vi "buscaclip.vi"(0 "input cluster":T1, 1 "Channels values 2":i32[](array[numeric]), 2 "vclip":i32[](array[numeric]), 5 "Channels init":i32[](array[numeric])=[2000], 7 "Boolean":bool, 9 "%desviacio":dbl=5.0, 11 "error out 2":errorcluster, 12 "Number points":i32, 13 "slope":dbl) -> (4 "slope 2":dbl, 6 "vclip 2":i32[](array[numeric]), 10 "XY Graph 2":cluster{dbl[], "Best Linear Fit":dbl[]}[](graph), 15 "error out":errorcluster)   [LabVIEW 2009]
uses:
  <vilib>/Utility/NIReport.llb/NI_report.lvclass
  <vilib>/Analysis/NI_AALPro.lvlib
panel:
  out "XY Graph 4":cluster{dbl[], "Best Linear Fit":dbl[]}(graph)
  out "XY Graph 3":cluster{dbl[], i32[]}(graph)
  in  "L1  50% invented":dbl[][](array[numeric])
  in  "L1 min invented":i32[](array[numeric])=[242, 504, 1031, 2128, 3263, 4418, 5634, 6888]
  out "XY Graph":cluster{"Y":dbl[], "Y":dbl[]}[](graph)
  out "L1  50%":dbl[][](array[numeric])=[[182.05332645693656, 181.0458957661739, 182.31328051706822, 182.44384615384615, 179.9591580860661, 183.67138786049767, 183.0415079653926], [383.1443079334591, 380.3408546343534, 383.09068068207546, 382.9081242164992, 377.8888565224893, 386.4745006061593, 384.33733278296165], [789.794916143154, 783.9334435523022, 789.880331635444, 788.1638578058222, 779.1397265900023, 796.380113600458, 792.3805482207972], [1637.2849189817332, 1624.3008579976345, 1635.9791868307739, 1633.4037928039274, 1613.351662874732, 1647.9524154468106, 1640.5214046384517], [2513.43820756283, 2496.681867952526, 2512.120672224883, 2508.5174246445135, 2478.2432072662637, 2532.0838659445626, 2519.7319162836616], [4350.429616233692, 4325.797863663112, 4346.430175185175, 4343.835753463216, 4286.1263991243895, 4381.02010040906, 4360.577157137679], [5321.96395522116, 5291.780098348377, 5317.9835218197695, 5305.673007498198, 5228.362955923682, 5348.7398745375585, 5316.2612416656], [6878.716199794284, 6844.2297782699125, 6886.512941570447, 6849.728580417201, 6743.132495285984, 6910.301756503628, 6900.4988799604525]]
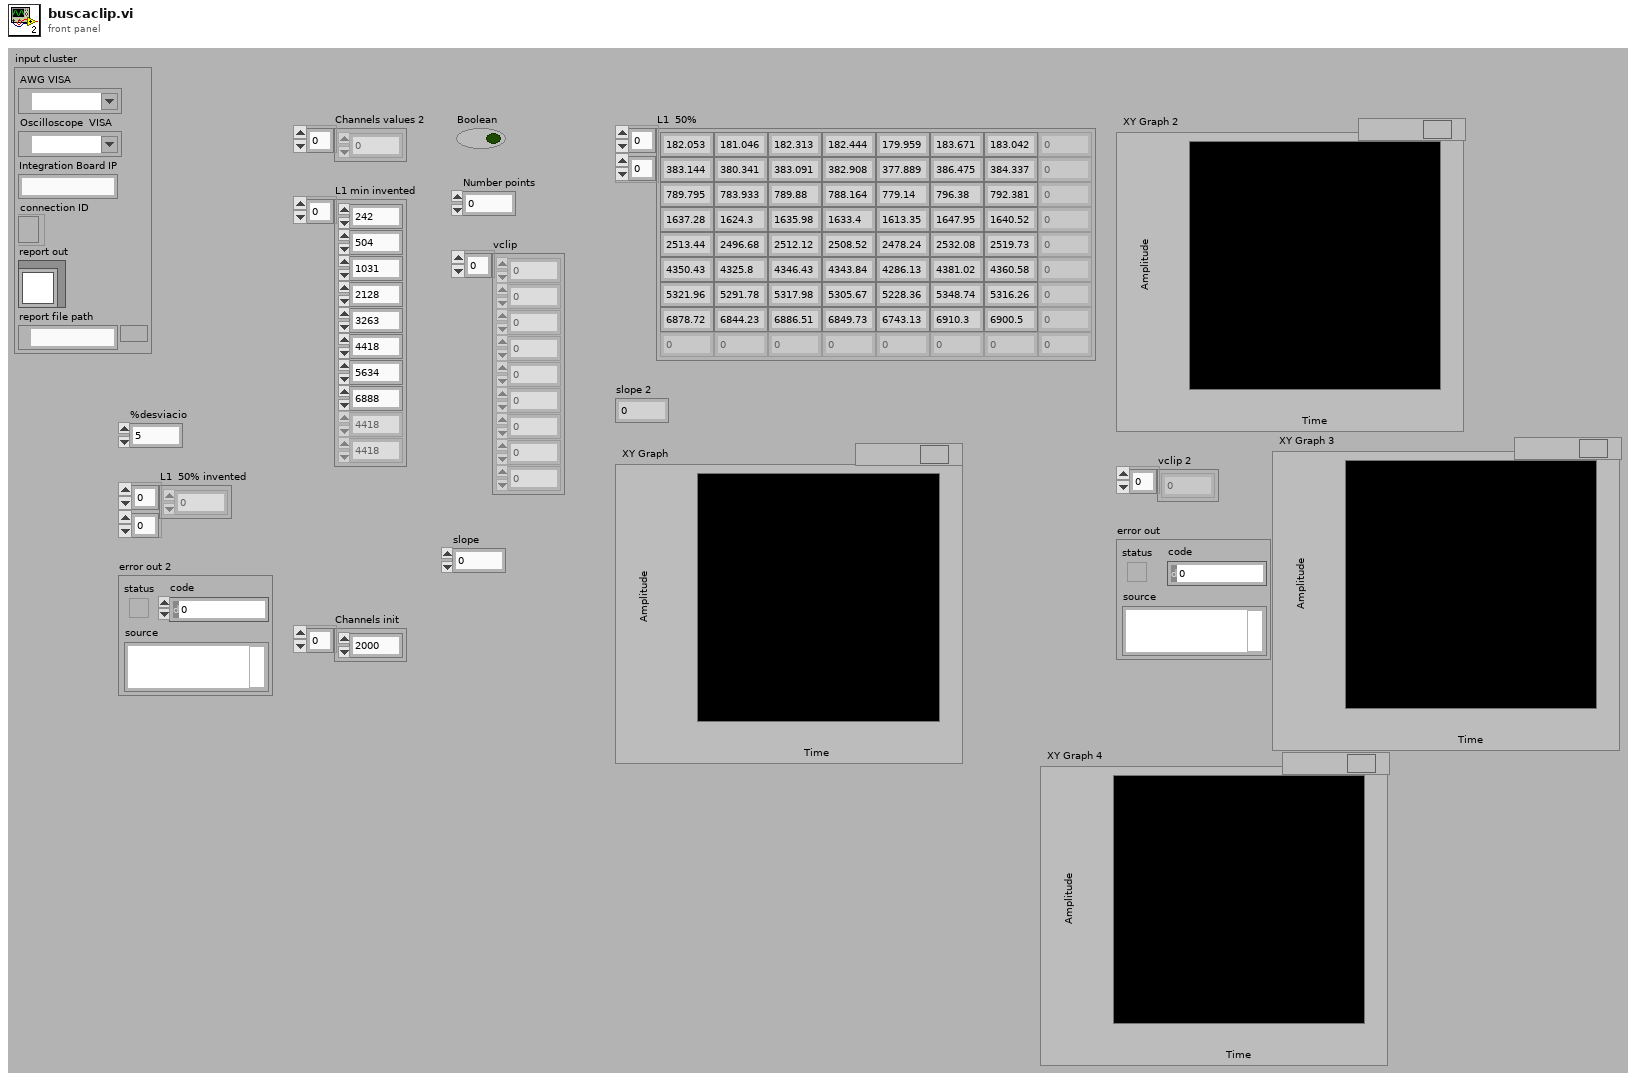
[diagram p1: front panel]
types:
  T1 = cluster{"AWG VISA":refnum<visa-resource-name>, "Oscilloscope  VISA ":refnum<visa-resource-name>, "Integration Board IP":string, "connection ID":refnum<k5>, "report out":refnum<class "NI_report.lvclass">, "report file path":path}
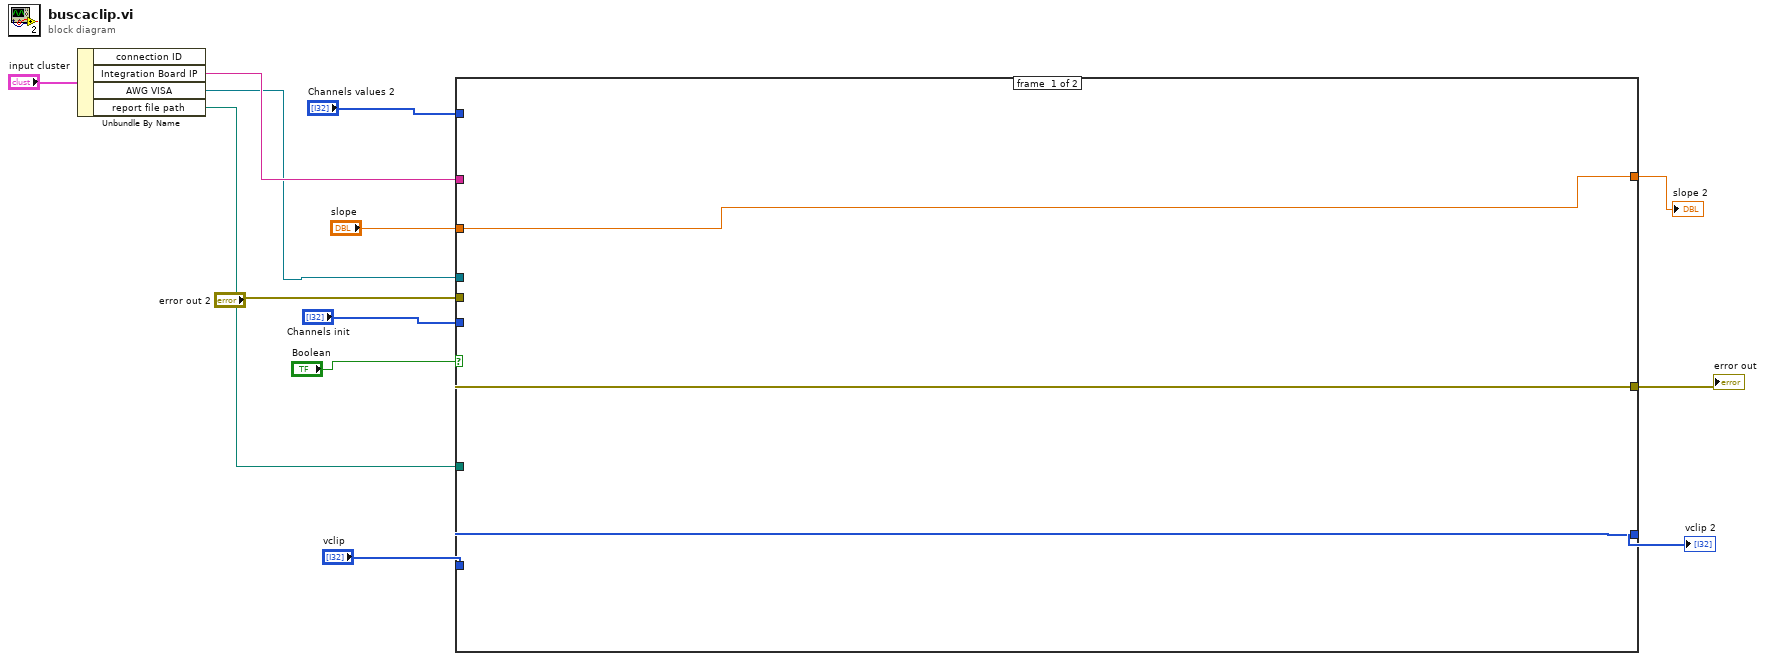
[diagram p0: block diagram]
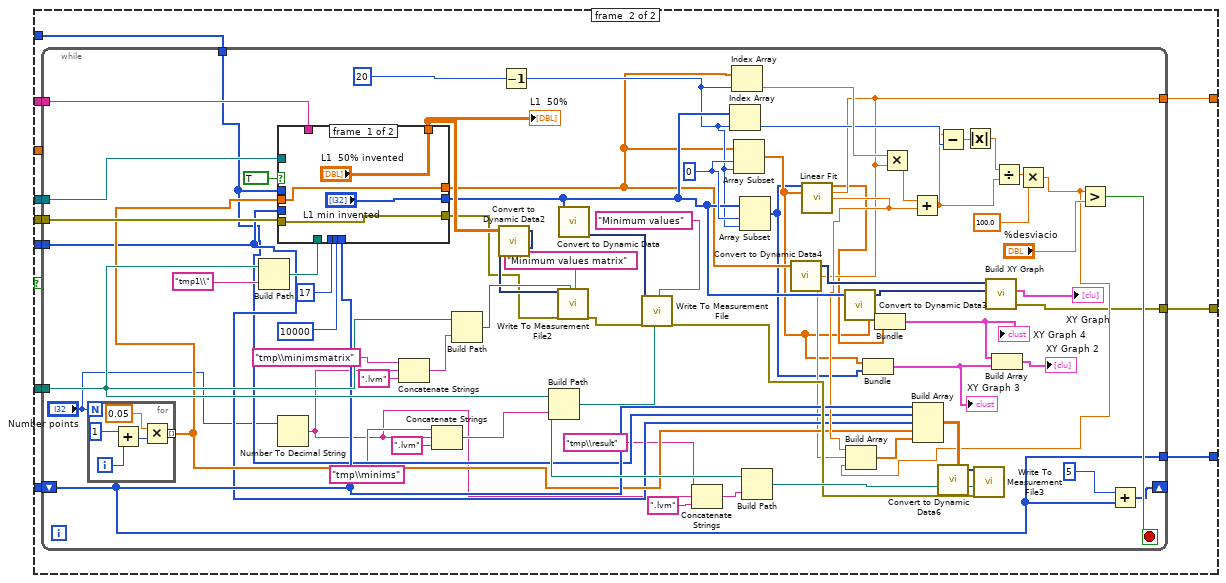
[diagram p2: hidden frame]
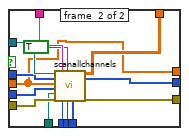
[diagram p3: hidden frame]
diagram:
  n1 = Unbundle By Name("input cluster") -> ("Integration Board IP"=w4:string, "AWG VISA"=w3:refnum<visa-resource-name>, "report file path"=w2:path)  [unwired: 1 out]
  n2 = case shown="True" "Boolean" {
    tunnel: "error out 2" -> [w14 w26]
    tunnel: w3 -> [_ w25]
    tunnel: w4 -> [_ w24]
    tunnel: w2 -> [_ w23]
    tunnel: [w15 w22] -> w11
    tunnel: [w16 w21] -> w7
    tunnel: "vclip" -> [w16 w20]
    tunnel: "Channels init" -> [_ w19]
    tunnel: "Channels values 2" -> [_ w18]
    tunnel: "slope" -> [w15 _]
    tunnel: [w14 w17] -> w13
    frame #0 {
    }
    frame #1 {
      n3 = while {
        tunnel: w26 -> [w91]
        tunnel: w25 -> [w90]
        tunnel: w24 -> [w89]
        tunnel: w23 -> [w62]
        shift-right: [w63] -> _
        shift-left: w20 -> [w59]
        tunnel: [w49] -> w22
        tunnel: [w59] -> w21
        tunnel: w19 -> [w51]
        tunnel: w18 -> [w50]
        tunnel: [w38] -> w17
        stop <- w73 stop-if-true
        w79 = 0 ("length")
        n4 = for {
          N: "Number points" -> [_]
          tunnel: [w95] -> w53 mode=indexing
          i -> [w99]
          n5 = Add(x=1, y=w99) -> (x+y=w97:i32)
          n6 = Multiply(x=0.05 ("y"), y=w97) -> (x*y=w95:dbl)
        }
        n7 = Build Path(base path=w62, name or relative path="tmp1\\") -> (appended path=w87:path)
        n8 = case shown="True" TRUE {
          tunnel: [w103 w117] -> w81
          tunnel: w91 -> [w103 w116]
          tunnel: w90 -> [_ w115]
          tunnel: w89 -> [_ w114]
          tunnel: w51 -> [_ w113]
          tunnel: w53 -> [w100 w104]
          tunnel: w50 -> [_ w112]
          tunnel: 17 ("Value") -> [_ w111]
          tunnel: 10000 ("Value") -> [_ w110]
          tunnel: ["L1 min invented" w108] -> w65
          tunnel: w87 -> [_ w107]
          tunnel: w59 -> [_ w106]
          tunnel: ["L1  50% invented" w105] -> w83
          tunnel: [w100 w104] -> w33
          frame #0 {
          }
          frame #1 {
            n9 = call "scanallchannels.vi"("VISA resource name out"=w115, "nm ch"=w112, "Voltages values"=w104, "Init ch value"=w113, "base path"=w107, "error in"=w116, "Integration Board IP"=w114, "L1 Address"=w111, "Save test data"=TRUE, "Ch burst"=w110, "vclip"=w106) -> ("L1  50%"=w105:dbl[][], "L1 min values"=w108:i32[], "error out"=w117:errorcluster)  [unwired: 6 in]
          }
        }
        "L1  50%" <- w83
        n10 = Number To Decimal String(number="Number points") -> (decimal integer string=w41:string)  [unwired: 1 in]
        n11 = Concatenate Strings("tmp\\minimsmatrix" ("name or relative path"), w41, ".lvm" ("string")) -> (w43:string)
        n12 = Concatenate Strings("tmp\\minims" ("name or relative path"), w41, ".lvm" ("string")) -> (w44:string)
        n13 = Build Path(base path=w62, name or relative path=w43) -> (appended path=w84:path)
        n14 = call "Convert to Dynamic Data2"("2D Array"=w83) -> ("Dynamic Data Type"=w82:dynamicdata)  [unwired: 3 in]
        n15 = Decrement(x=20) -> (x-1=w52:i32)
        n16 = Build Path(base path=w62, name or relative path=w44) -> (appended path=w92:path)
        n17 = call "Write To Measurement File2"("Signals"=w82, "error in (no error)"=w81, "Filename"=w84, "Comment"="Minimum values matrix") -> ("error out"=w80:errorcluster)  [unwired: 13 in, 2 out]
        n18 = call "Convert to Dynamic Data"("Array"=w65) -> ("Dynamic Data Type"=w94:dynamicdata)  [unwired: 3 in]
        n19 = call "Write To Measurement File"("Signals"=w94, "error in (no error)"=w80, "Filename"=w92, "Comment"="Minimum values") -> ("error out"=w60:errorcluster)  [unwired: 13 in, 2 out]
        n20 = Concatenate Strings("tmp\\result" ("name or relative path"), w41, ".lvm" ("string")) -> (w39:string)
        n21 = Index Array(array=w65, index=w52) -> (element=w68:i32)
        n22 = Index Array(array=w33, index=w52) -> (element=w78:dbl)
        n23 = Array Subset(array=w33, index=w79, length=w52) -> (w31:dbl[])
        n24 = Array Subset(array=w65, index=w79, length=w52) -> (w30:i32[])
        n25 = Build Path(base path=w62, name or relative path=w39) -> (appended path=w61:path)
        n26 = call "Convert to Dynamic Data4"("Array"=w33) -> ("Dynamic Data Type"=w66:dynamicdata)  [unwired: 3 in]
        n27 = call <vilib>:"Linear Fit.vi"("Y"=w30, "X"=w31) -> ("Best Linear Fit"=w32:dbl[], "slope"=w49:dbl, "intercept"=w58:dbl)  [unwired: 9 in, 2 out]
        n28 = call "Convert to Dynamic Data3"("Array"=w65) -> ("Dynamic Data Type"=w67:dynamicdata)  [unwired: 3 in]
        n29 = Bundle(w31, w30) -> (w27:cluster{dbl[], i32[]})  [unwired: 1 in]
        "XY Graph 3" <- w27
        n30 = Bundle(w31, "Best Linear Fit"=w32) -> (w29:cluster{dbl[], "Best Linear Fit":dbl[]})  [unwired: 1 in]
        "XY Graph 4" <- w29
        n31 = Multiply(x=w78, y=w49) -> (x*y=w77:dbl)
        n32 = Add(x=w77, y=w58) -> (x+y=w64:dbl)
        n33 = Subtract(x=w64, y=w68) -> (x-y=w76:dbl)
        n34 = Absolute Value(x=w76) -> (abs(x)=w75:dbl)
        n35 = call "Build XY Graph"("Y Input"=w67, "X Input"=w66) -> ("error out"=w38:errorcluster, "XY Graph"=→"XY Graph":cluster{"Y":dbl[], "Y":dbl[]}[])  [unwired: 8 in]
        n36 = Build Array(w29, w27) -> (→"XY Graph 2":cluster{dbl[], "Best Linear Fit":dbl[]}[])
        n37 = Divide(x=w75, y=w64) -> (x/y=w71:dbl)
        n38 = Multiply(x=w71, y=100.0) -> (x*y=w54:dbl)
        n39 = Build Array(w58, w49, w54) -> (w57:dbl[])
        n40 = Build Array(w59, w50, w51, w53, w57) -> (w56:dbl[][])
        n41 = call "Convert to Dynamic Data6"("2D Array"=w56) -> ("Dynamic Data Type"=w55:dynamicdata)  [unwired: 3 in]
        n42 = call "Write To Measurement File3"("Signals"=w55, "error in (no error)"=w60, "Filename"=w61) -> ()  [unwired: 14 in, 3 out]
        n43 = Greater?(x=w54, y="%desviacio") -> (0:w73:bool)
        n44 = Add(x=5, y=w59) -> (x+y=w63:i32[])
      }
    }
  }
  "error out" <- w13
  "slope 2" <- w11
  "vclip 2" <- w7
